vi "Begin.vi"(8 "error in":errorcluster) -> (0 "error out":errorcluster)   [LabVIEW 2020]
doc: "Called before other user functions, this VI is expected to open initial I/O refnums, load in file data, and do all program initialization. Notice that the <B>error out</B> terminal is simply used for data flow. Wiring it to other structures or subVIs ensures that this VI runs first."
uses:
  <vilib>/Rock Robotics/WPI/DriverStation/WPI_DriverStationRobotMode2.ctl
  <vilib>/Rock Robotics/WPI/Joystick/WPI_JoystickDeviceEnum.ctl
  <vilib>/Rock Robotics/WPI/Solenoid/WPI_SolenoidChannel.ctl
  <vilib>/Rock Robotics/SystemInterfaces/DIO/FPGA_DIOPWMChannel.ctl
  <vilib>/Rock Robotics/SystemInterfaces/DIO/FPGA_DIOChannel.ctl
  <vilib>/Rock Robotics/WPI/Encoder/WPI_EncoderType.ctl
  <vilib>/Rock Robotics/WPI/SafetyOutput/WPI_SafetyOutputConfigMenu.ctl
  Robot Global Data.vi
  <vilib>/Rock Robotics/Network Tables/NT Write String Array.vi
  <vilib>/Rock Robotics/WPI/RobotDrive/WPI_RobotDriveOpen4MotorWithExistingMotors.vi
  <vilib>/Rock Robotics/WPI/Solenoid/WPI_SolenoidOpenDouble.vi
  <vilib>/Rock Robotics/WPI/Counter/WPI_CounterDigitalInputToDigitalSource.vi
  <vilib>/Rock Robotics/WPI/RobotDrive/WPI_RobotDriveOpen2MotorWithVictorSPX.vi
  <vilib>/Rock Robotics/SystemInterfaces/spilib/spi_bus.ctl
  <vilib>/Rock Robotics/WPI/Gyro/WPI_GyroXRS450_SPI_Open.vi
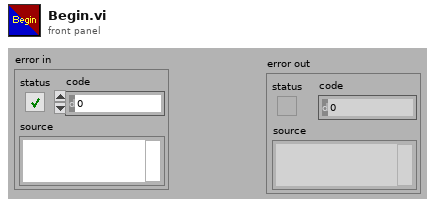
[diagram p1: front panel]
types:
  T1 = typedef "WPI_EncoderType.ctl" = enum16{"1x", "2x", "4x"}
  T2 = typedef "FPGA_DIOChannel.ctl" = enum8{"DIO 0", "DIO 1", "DIO 2", "DIO 3", "DIO 4", "DIO 5", "DIO 6", "DIO 7", "DIO 8", "DIO 9", "DIO MXP 0", "DIO MXP 1", "DIO MXP 2", "DIO MXP 3", "DIO MXP 4", "DIO MXP 5", "DIO MXP 6", "DIO MXP 7", "DIO MXP 8", "DIO MXP 9", "DIO MXP 10", "DIO MXP 11", "DIO MXP 12", "DIO MXP 13", "DIO MXP 14", "DIO MXP 15", "SPI Port CS1", "SPI Port CS2", "SPI Port CS3", "SPI Port MISO", "SPI Port MOSI", "Invalid"}
  T3 = typedef "FPGA_DIOPWMChannel.ctl" = enum8{"PWM 0", "PWM 1", "PWM 2", "PWM 3", "PWM 4", "PWM 5", "PWM 6", "PWM 7", "PWM 8", "PWM 9", "PWM MXP 0", "PWM MXP 1", "PWM MXP 2", "PWM MXP 3", "PWM MXP 4", "PWM MXP 5", "PWM MXP 6", "PWM MXP 7", "PWM MXP 8", "PWM MXP 9", "Invalid"}
  T4 = typedef "WPI_SolenoidChannel.ctl" = enum8{"Solenoid 0", "Solenoid 1", "Solenoid 2", "Solenoid 3", "Solenoid 4", "Solenoid 5", "Solenoid 6", "Solenoid 7", "Solenoid 8", "Solenoid 9", "Solenoid 10", "Solenoid 11", "Solenoid 12", "Solenoid 13", "Solenoid 14", "Solenoid 15", "Invalid"}
  T5 = typedef "WPI_JoystickDeviceEnum.ctl" = enum16{"USB 0", "USB 1", "USB 2", "USB 3", "USB 4", "USB 5"}
  T6 = typedef "WPI_DriverStationRobotMode2.ctl" = enum16{"Autonomous Disabled", "Autonomous Enabled", "Teleop Disabled", "Teleop Enabled", "Disconnected", "Finish", "Test Disabled", "Test Enabled", "Emergency Stopped"}
  T7 = typedef "WPI_MotorControlDeviceRef.ctl" = cluster{"DeviceStatus":errorcluster, "Type":T8, "PWM":cluster{"PWM Channel":T3, "DeadBand":T9}, "CAN":cluster{"Device Number":u8, "SetOutput VI Ref":variant, "GetOutput VI Ref":variant, "Enable VI Ref":variant, "Disable VI Ref":variant, "Data":variant}, "Invert":bool, "DIO PWM":cluster{"PWM \"Enable\" Channel":T3, "DIOChannel":T2, "PWM Rate":dbl}}
  T8 = typedef "WPI_MotorControlType.ctl" = enum16{"PWM", "CAN", "DIO PWM"}
  T9 = typedef "WPI_PWMDeadband.ctl" = cluster{"Name":string, "maxPositivePwm":i32, "minPositivePwm":i32, "centerPwm":i32, "maxNegativePwm":i32, "minNegativePwm":i32, "angularRange":u16}
  T10 = typedef "spi_bus.ctl" = enum16{"SPI On-Board, CS0", "SPI On-Board, CS1", "SPI On-Board, CS2", "SPI On-Board, CS3", "SPI MXP", "Invalid"}
  T11 = typedef "WPI_GyroDevRef.ctl" = cluster{"DevStatus":errorcluster, "Analog Channel":T12, "Gain (VoltsPerDegree/Second)":dbl, "Gyro Type":enum16{"Analog", "XRS450"}, "Handle":i32, "SPI Bus":T10, "Device Found":bool, "Sample Rate":dbl, "Calibrate On Open":bool, "Offset":dbl}
  T12 = typedef "FPGA_AIChannel.ctl" = enum8{"AI 0", "AI 1", "AI 2", "AI 3", "AI MXP 0", "AI MXP 1", "AI MXP 2", "AI MXP 3", "Invalid"}
  T13 = typedef "WPI_ServoDeviceRef.ctl" = cluster{"DeviceStatus":errorcluster, "PWM Channel":T3, "DeadBand":T9}
  T14 = typedef "WPI_JoystickDevRef.ctl" = cluster{"Device":T5}
  T15 = typedef "WPI_DigitalInputDevRef.ctl" = cluster{"DevStatus":errorcluster, "DIO Channel":T2}
  T16 = typedef "FPGA_CounterEncoderSourceConvertionLVSourceType.ctl" = cluster{"DevStatus":errorcluster, "AnalogTriggerMode?":bool, "DigitalMode":cluster{"DIO Channel":T17}, "AnalogTriggerMode":cluster{"AnalogTriggerIndex":T18, "OutputType":T19}}
  T17 = typedef "FPGA_DIODigitalSourceChannel.ctl" = enum8{"DIO 0", "DIO 1", "DIO 2", "DIO 3", "DIO 4", "DIO 5", "DIO 6", "DIO 7", "DIO 8", "DIO 9", "DIO MXP 0", "DIO MXP 1", "DIO MXP 2", "DIO MXP 3", "DIO MXP 4", "DIO MXP 5", "DIO MXP 6", "DIO MXP 7", "DIO MXP 8", "DIO MXP 9", "DIO MXP 10", "DIO MXP 11", "DIO MXP 12", "DIO MXP 13", "DIO MXP 14", "DIO MXP 15", "SPI Port CS1", "SPI Port CS2", "SPI Port CS3", "SPI Port MISO", "SPI Port MOSI", "Disabled"}
  T18 = typedef "FPGA_AnalogTriggerIndex.ctl" = enum8{"Trig 0", "Trig 1", "Trig 2", "Trig 3", "Trig 4", "Trig 5", "Trig 6", "Trig 7", "Invalid"}
  T19 = typedef "FPGA_AnalogTriggerOutType.ctl" = enum16{"InWindow", "TriggerState", "Rising", "Falling"}
  T20 = typedef "WPI_EncoderDevRef.ctl" = cluster{"DevStatus":errorcluster, "EncoderIndex":T21, "CounterIndex":T22, "DistancePerCount":dbl, "Decoding Type":T1}
  T21 = typedef "FPGA_EncoderIdx.ctl" = enum8{"Enc 0", "Enc 1", "Enc 2", "Enc 3", "Enc 4", "Enc 5", "Enc 6", "Enc 7", "Invalid"}
  T22 = typedef "FPGA_CounterCtrSystemIndex.ctl" = enum8{"Ctr 0", "Ctr 1", "Ctr 2", "Ctr 3", "Ctr 4", "Ctr 5", "Ctr 6", "Ctr 7", "Invalid"}
  T23 = typedef "WPI_SafetyOutputConfigMenu.ctl" = enum16{"Enable", "Disable"}
  T24 = typedef "WPI_RobotDriveDevRef.ctl" = cluster{"DevStatus":errorcluster, "Motors[]":T7[], "Square Inputs":bool, "Max Output":dbl}
  T25 = typedef "WPI_SolenoidDevRef.ctl" = cluster{"DevStatus":errorcluster, "Pneumatics Control Module":u8, "Forward Solenoid Channel":T4, "Reverse Solenoid Channel":T4}
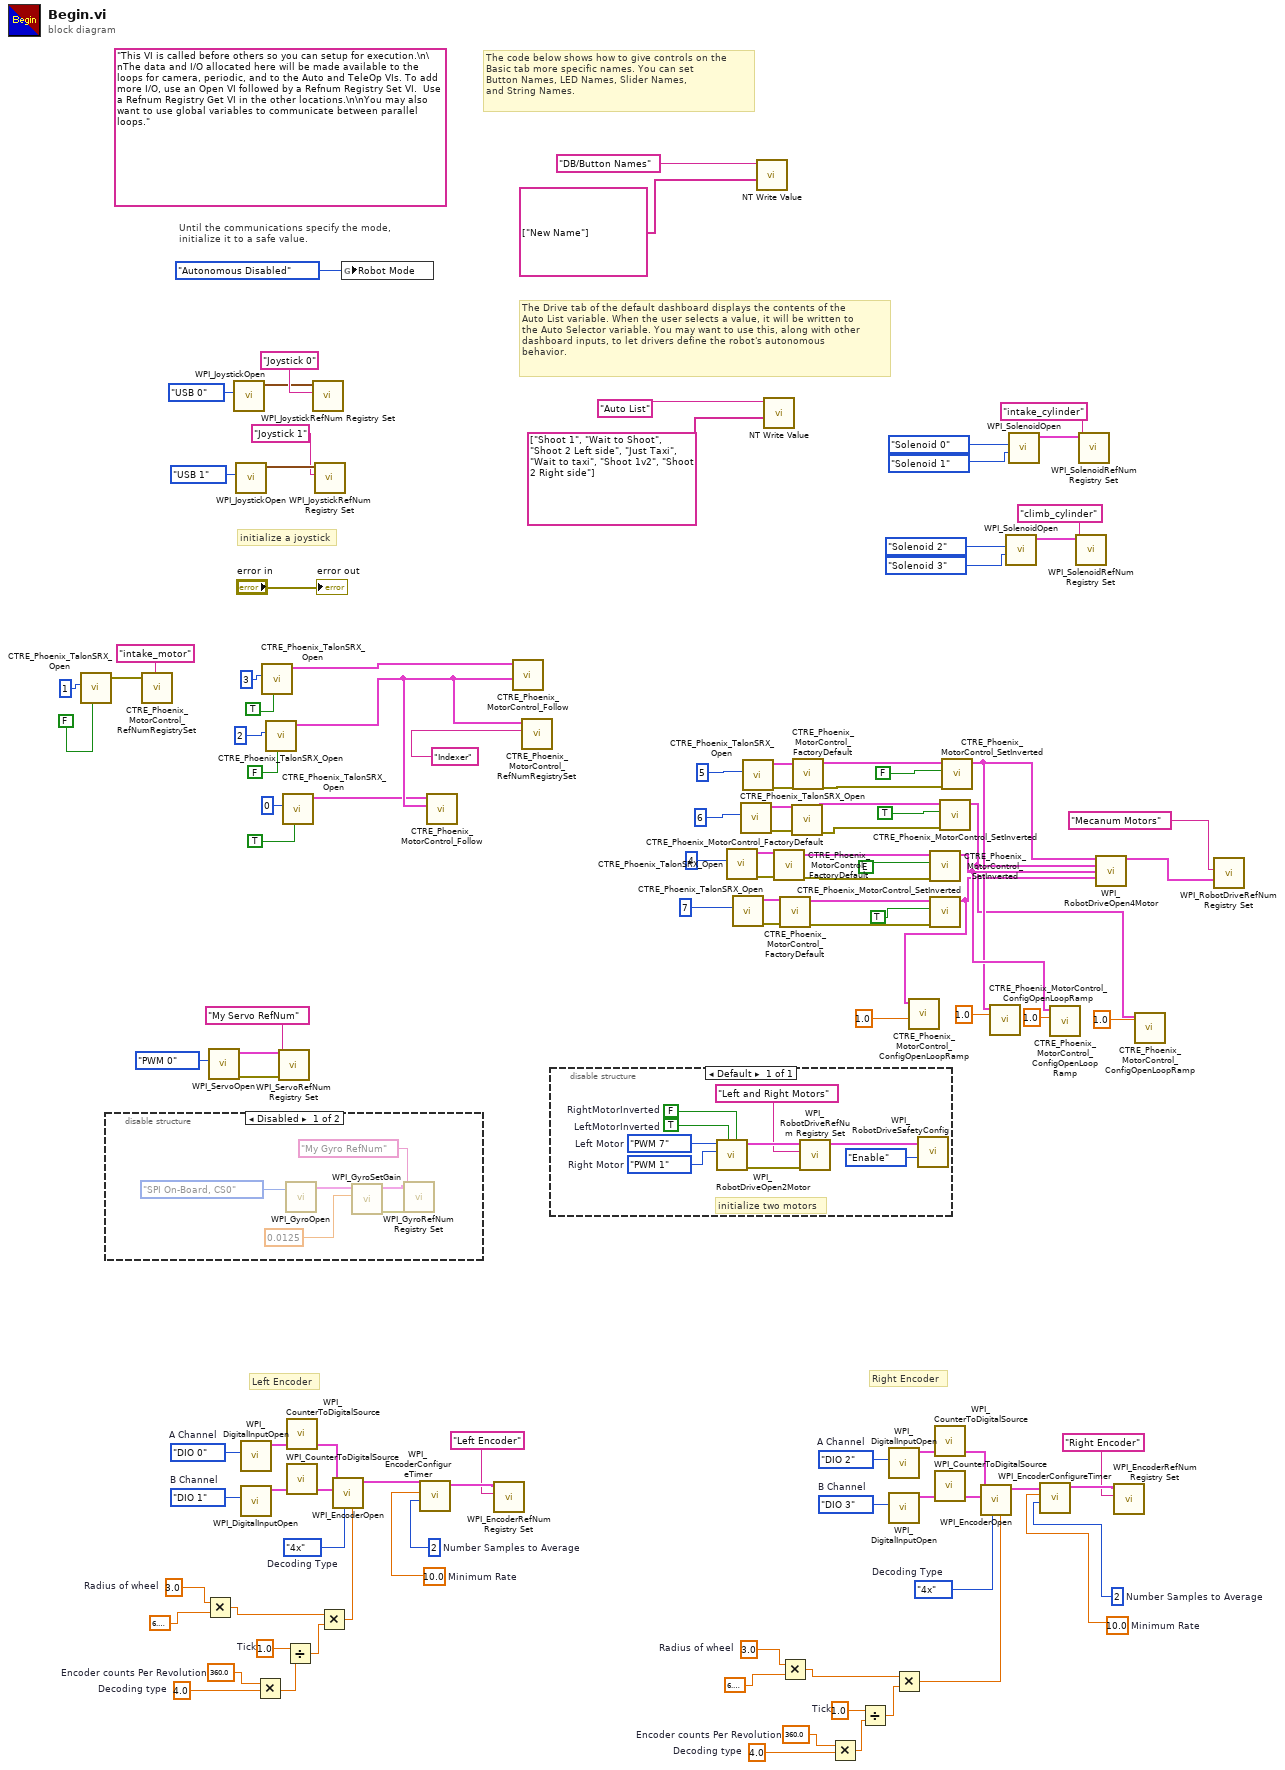
[diagram p0: block diagram]
diagram:
  w5 = u8 2  # Number Samples to Average
  w3 = 10.0  # Minimum Rate
  w9 = 3.0  # Radius of wheel
  w10 = 1.0  # Tick
  w13 = 360.0  # Encoder counts Per Revolution
  w14 = 4.0  # Decoding type
  w6 = WPI_EncoderType."4x"  # Decoding Type
  w1 = u8 2  # Number Samples to Average
  w15 = 10.0  # Minimum Rate
  w17 = 3.0  # Radius of wheel
  w19 = 1.0  # Tick
  w23 = 360.0  # Encoder counts Per Revolution
  w24 = 4.0  # Decoding type
  w2 = WPI_EncoderType."4x"  # Decoding Type
  w34 = FPGA_DIOChannel."DIO 3"  # B Channel
  w33 = FPGA_DIOChannel."DIO 2"  # A Channel
  w40 = FPGA_DIOChannel."DIO 1"  # B Channel
  w39 = FPGA_DIOChannel."DIO 0"  # A Channel
  (unwired) "This VI is called before others so you can setup for execution.\n\nThe data and I/O allocated here will be made available to the loops for camera, periodic, and to the Auto and TeleOp VIs. To add more I/O, use an Open VI followed by a Refnum Registry Set VI.  Use a Refnum Registry Get VI in the other locations.\n\nYou may also want to use global variables to communicate between parallel loops."
  # "Right Encoder"
  # "Left Encoder"
  # "The Drive tab of the default dashboard displays the contents of the\nAuto List variable. When the user selects a value, it will be written to\nthe Auto Selector variable. You may want to use this, along with other\ndashboard inputs, to let drivers define the robot's autonomous\nbehavior."
  # "The code below shows how to give controls on the\nBasic tab more specific names. You can set\nButton Names, LED Names, Slider Names,\nand String Names."
  # "initialize a joystick"
  # "Until the communications specify the mode,\ninitialize it to a safe value."
  n1 = call <vilib>:"CTRE_Phoenix_TalonSRX_Open.vi"("Invert"=FALSE, "Device Number"=u8 1) -> ("error out"=w79:errorcluster, "PhoenixMotorControlDevRef"=w78:T7)  [unwired: 8 in]
  n2 = disable-structure shown="Disabled" {
    frame Disabled {
      n3 = call-poly <vilib>:"WPI_GyroOpen.vi"("SPI Bus"=spi_bus."SPI On-Board, CS0") -> ("GyroDevRef"=w118:T11)  [unwired: 8 in, 2 out]
      n4 = call <vilib>:"WPI_GyroSetGain.vi"("Gain (VoltsPerDegree/Second)"=0.0125, "GyroDevRef"=w118) -> ("error out"=w119:errorcluster, "GyroDevRef"=w117:T11)  [unwired: 8 in]
      n5 = call <vilib>:"WPI_GyroRefNum Registry Set.vi"("error in (no error)"=w119, "refnum name"="My Gyro RefNum", "GyroDevRef"=w117) -> ()  [unwired: 7 in, 2 out]
    }
    frame Enabled {
    }
  }
  n6 = call <vilib>:"CTRE_Phoenix_MotorControl_RefNumRegistrySet.vi"("error in (no error)"=w79, "refnum name"="intake_motor", "PhoenixMotorControlDevRef"=w78) -> ()  [unwired: 7 in, 2 out]
  n7 = Multiply(x=w17, y=6.283185307179586) -> (x*y=w18:dbl)
  n8 = call <vilib>:"WPI_ServoOpen.vi"("PWM Channel"=FPGA_DIOPWMChannel."PWM 0") -> ("error out"=w44:errorcluster, "ServoDeviceRef"=w45:T13)  [unwired: 9 in]
  n9 = call <vilib>:"WPI_JoystickOpen.vi"("JoystickDevice"=WPI_JoystickDeviceEnum."USB 0") -> ("JoystickDevRef"=w112:T14)  [unwired: 10 in]
  n10 = call <vilib>:"WPI_JoystickOpen.vi"("JoystickDevice"=WPI_JoystickDeviceEnum."USB 1") -> ("JoystickDevRef"=w76:T14)  [unwired: 10 in]
  n11 = call <vilib>:"WPI_DigitalInputOpen.vi"("DIO Channel"=w39) -> ("DigitalInputDevRef"=w37:T15)  [unwired: 1 in, 9 out]
  n12 = call <vilib>:"WPI_DigitalInputOpen.vi"("DIO Channel"=w40) -> ("DigitalInputDevRef"=w38:T15)  [unwired: 1 in, 9 out]
  n13 = Multiply(x=w23, y=w24) -> (x*y=w20:dbl)
  n14 = call <vilib>:"CTRE_Phoenix_TalonSRX_Open.vi"("Invert"=TRUE, "Device Number"=u8 3) -> ("PhoenixMotorControlDevRef"=w67:T7)  [unwired: 8 in, 1 out]
  n15 = call <vilib>:"CTRE_Phoenix_TalonSRX_Open.vi"("Invert"=FALSE, "Device Number"=u8 2) -> ("PhoenixMotorControlDevRef"=w48:T7)  [unwired: 8 in, 1 out]
  n16 = call <vilib>:"WPI_ServoRefNum Registry Set.vi"("error in (no error)"=w44, "refnum name"="My Servo RefNum", "ServoDeviceRef"=w45) -> ()  [unwired: 7 in, 2 out]
  n17 = call <vilib>:"CTRE_Phoenix_TalonSRX_Open.vi"("Invert"=TRUE, "Device Number"=u8 0) -> ("PhoenixMotorControlDevRef"=w47:T7)  [unwired: 8 in, 1 out]
  n18 = Divide(x=w19, y=w20) -> (x/y=w21:dbl)
  n19 = call-poly <vilib>:"WPI_CounterToDigitalSource.vi"("DigitalInputDevRef"=w37) -> ("Digital Source"=w41:T16)  [unwired: 6 out]
  n20 = call-poly <vilib>:"WPI_CounterToDigitalSource.vi"("DigitalInputDevRef"=w38) -> ("Digital Source"=w42:T16)  [unwired: 6 out]
  n21 = call <vilib>:"WPI_JoystickRefNum Registry Set.vi"("refnum name"="Joystick 0", "JoystickDevRef"=w112) -> ()  [unwired: 8 in, 2 out]
  n22 = call <vilib>:"WPI_JoystickRefNum Registry Set.vi"("refnum name"="Joystick 1", "JoystickDevRef"=w76) -> ()  [unwired: 8 in, 2 out]
  n23 = Multiply(x=w18, y=w21) -> (x*y=w22:dbl)
  n24 = call <vilib>:"WPI_EncoderOpen.vi"("DistancePerCount"=w22, "Decoding Type"=w2, "BSource"=w42, "ASource"=w41) -> ("EncoderDevRef"=w30:T20)  [unwired: 6 in, 1 out]
  n25 = global write "Robot Global Data.vi" "Robot Mode"(WPI_DriverStationRobotMode2."Autonomous Disabled" ("Robot Mode")) -> ()
  n26 = call <vilib>:"WPI_EncoderConfigureTimer.vi"("Number Samples to Average"=w1, "Minimum Rate"=w15, "EncoderDevRef"=w30) -> ("EncoderDevRef"=w29:T20)  [unwired: 7 in, 1 out]
  n27 = call <vilib>:"CTRE_Phoenix_MotorControl_Follow.vi"("Master Controller to Follow"=w48, "PhoenixMotorControlDevRef"=w47) -> ()  [unwired: 8 in, 2 out]
  n28 = call <vilib>:"WPI_EncoderRefNum Registry Set.vi"("refnum name"="Left Encoder", "EncoderDevRef"=w29) -> ()  [unwired: 8 in, 2 out]
  n29 = call <vilib>:"CTRE_Phoenix_MotorControl_Follow.vi"("Master Controller to Follow"=w48, "PhoenixMotorControlDevRef"=w67) -> ()  [unwired: 8 in, 2 out]
  n30 = call <vilib>:"CTRE_Phoenix_MotorControl_RefNumRegistrySet.vi"("refnum name"="Indexer", "PhoenixMotorControlDevRef"=w48) -> ()  [unwired: 8 in, 2 out]
  n31 = disable-structure shown="Default" {
    frame Enabled {
      w123 = FPGA_DIOPWMChannel."PWM 1"  # Right Motor
      w124 = FPGA_DIOPWMChannel."PWM 7"  # Left Motor
      w128 = TRUE  # LeftMotorInverted
      w129 = FALSE  # RightMotorInverted
      # "initialize two motors"
      n32 = call-poly <vilib>:"WPI_RobotDriveOpen2Motor.vi"("Right Motor Inverted"=w129, "Left Motor Inverted"=w128, "Right Motor"=w123, "Left Motor"=w124) -> ("error out"=w125:errorcluster, "RobotDriveDevRef"=w127:T24)  [unwired: 1 in, 5 out]
      n33 = call <vilib>:"WPI_RobotDriveRefNum Registry Set.vi"("error in (no error)"=w125, "refnum name"="Left and Right Motors", "RobotDriveDevRef"=w127) -> ("RobotDriveDevRef"=w122:T24)  [unwired: 1 in, 7 out]
      n34 = call <vilib>:"WPI_RobotDriveSafetyConfig.vi"("mode"=WPI_SafetyOutputConfigMenu."Enable", "RobotDriveDevRef"=w122) -> ()  [unwired: 8 in, 2 out]
    }
  }
  n35 = call <vilib>:"CTRE_Phoenix_TalonSRX_Open.vi"("Device Number"=u8 4) -> ("error out"=w104:errorcluster, "PhoenixMotorControlDevRef"=w105:T7)  [unwired: 9 in]
  n36 = call <vilib>:"CTRE_Phoenix_TalonSRX_Open.vi"("Device Number"=u8 7) -> ("error out"=w94:errorcluster, "PhoenixMotorControlDevRef"=w95:T7)  [unwired: 9 in]
  n37 = call <vilib>:"CTRE_Phoenix_TalonSRX_Open.vi"("Device Number"=u8 6) -> ("error out"=w98:errorcluster, "PhoenixMotorControlDevRef"=w99:T7)  [unwired: 9 in]
  n38 = call <vilib>:"CTRE_Phoenix_TalonSRX_Open.vi"("Device Number"=u8 5) -> ("error out"=w91:errorcluster, "PhoenixMotorControlDevRef"=w101:T7)  [unwired: 9 in]
  n39 = call-poly <vilib>:"NT Write Value.vi"("String Array"=string[] ["New Name"], "Name"="DB/Button Names") -> ()  [unwired: 9 in, 1 out]
  n40 = call-poly <vilib>:"NT Write Value.vi"("String Array"=string[] ["Shoot 1", "Wait to Shoot", "Shoot 2 Left side", "Just Taxi", "Wait to taxi", "Shoot 1v2", "Shoot 2 Right side"], "Name"="Auto List") -> ()  [unwired: 9 in, 1 out]
  n41 = call <vilib>:"CTRE_Phoenix_MotorControl_FactoryDefault.vi"("error in"=w104, "PhoenixMotorControlDevRef"=w105) -> ("error out"=w102:errorcluster, "PhoenixMotorControlDevRef"=w103:T7)  [unwired: 8 in]
  n42 = call <vilib>:"CTRE_Phoenix_MotorControl_FactoryDefault.vi"("error in"=w94, "PhoenixMotorControlDevRef"=w95) -> ("error out"=w92:errorcluster, "PhoenixMotorControlDevRef"=w93:T7)  [unwired: 8 in]
  n43 = Multiply(x=w9, y=6.283185307179586) -> (x*y=w4:dbl)
  n44 = call <vilib>:"CTRE_Phoenix_MotorControl_FactoryDefault.vi"("error in"=w98, "PhoenixMotorControlDevRef"=w99) -> ("error out"=w96:errorcluster, "PhoenixMotorControlDevRef"=w97:T7)  [unwired: 8 in]
  n45 = call <vilib>:"CTRE_Phoenix_MotorControl_FactoryDefault.vi"("PhoenixMotorControlDevRef"=w101) -> ("PhoenixMotorControlDevRef"=w100:T7)  [unwired: 9 in, 1 out]
  n46 = Multiply(x=w13, y=w14) -> (x*y=w11:dbl)
  n47 = Divide(x=w10, y=w11) -> (x/y=w12:dbl)
  n48 = call <vilib>:"WPI_DigitalInputOpen.vi"("DIO Channel"=w33) -> ("DigitalInputDevRef"=w31:T15)  [unwired: 1 in, 9 out]
  n49 = call <vilib>:"WPI_DigitalInputOpen.vi"("DIO Channel"=w34) -> ("DigitalInputDevRef"=w32:T15)  [unwired: 1 in, 9 out]
  n50 = Multiply(x=w4, y=w12) -> (x*y=w7:dbl)
  n51 = call <vilib>:"CTRE_Phoenix_MotorControl_SetInverted.vi"("error in (no error)"=w102, "Invert?"=FALSE, "PhoenixMotorControlDevRef"=w103) -> ("PhoenixMotorControlDevRef"=w58:T7)  [unwired: 7 in, 1 out]
  n52 = call <vilib>:"CTRE_Phoenix_MotorControl_SetInverted.vi"("error in (no error)"=w92, "Invert?"=TRUE, "PhoenixMotorControlDevRef"=w93) -> ("PhoenixMotorControlDevRef"=w51:T7)  [unwired: 7 in, 1 out]
  n53 = call <vilib>:"CTRE_Phoenix_MotorControl_ConfigOpenLoopRamp.vi"("secondsFromNeutralToFull"=1.0, "PhoenixMotorControlDevRef"=w51) -> ()  [unwired: 8 in, 2 out]
  n54 = call-poly <vilib>:"WPI_CounterToDigitalSource.vi"("DigitalInputDevRef"=w31) -> ("Digital Source"=w35:T16)  [unwired: 6 out]
  n55 = call-poly <vilib>:"WPI_CounterToDigitalSource.vi"("DigitalInputDevRef"=w32) -> ("Digital Source"=w36:T16)  [unwired: 6 out]
  n56 = call <vilib>:"CTRE_Phoenix_MotorControl_SetInverted.vi"("error in (no error)"=w96, "Invert?"=TRUE, "PhoenixMotorControlDevRef"=w97) -> ("PhoenixMotorControlDevRef"=w52:T7)  [unwired: 7 in, 1 out]
  n57 = call <vilib>:"CTRE_Phoenix_MotorControl_SetInverted.vi"("error in (no error)"=w91, "Invert?"=FALSE, "PhoenixMotorControlDevRef"=w100) -> ("PhoenixMotorControlDevRef"=w57:T7)  [unwired: 7 in, 1 out]
  n58 = call <vilib>:"WPI_EncoderOpen.vi"("DistancePerCount"=w7, "Decoding Type"=w6, "BSource"=w36, "ASource"=w35) -> ("EncoderDevRef"=w25:T20)  [unwired: 6 in, 1 out]
  n59 = call <vilib>:"CTRE_Phoenix_MotorControl_ConfigOpenLoopRamp.vi"("secondsFromNeutralToFull"=1.0, "PhoenixMotorControlDevRef"=w57) -> ()  [unwired: 8 in, 2 out]
  n60 = call-poly <vilib>:"WPI_SolenoidOpen.vi"("Reverse Solenoid Channel"=WPI_SolenoidChannel."Solenoid 3" ("Forward Solenoid Channel"), "Forward Solenoid Channel"=WPI_SolenoidChannel."Solenoid 2") -> ("SolenoidDevRef"=w65:T25)  [unwired: 8 in, 1 out]
  n61 = call-poly <vilib>:"WPI_SolenoidOpen.vi"("Reverse Solenoid Channel"=WPI_SolenoidChannel."Solenoid 1" ("Forward Solenoid Channel"), "Forward Solenoid Channel"=WPI_SolenoidChannel."Solenoid 0") -> ("SolenoidDevRef"=w62:T25)  [unwired: 8 in, 1 out]
  n62 = call <vilib>:"WPI_EncoderConfigureTimer.vi"("Number Samples to Average"=w5, "Minimum Rate"=w3, "EncoderDevRef"=w25) -> ("EncoderDevRef"=w27:T20)  [unwired: 7 in, 1 out]
  n63 = call <vilib>:"CTRE_Phoenix_MotorControl_ConfigOpenLoopRamp.vi"("secondsFromNeutralToFull"=1.0, "PhoenixMotorControlDevRef"=w58) -> ()  [unwired: 8 in, 2 out]
  n64 = call <vilib>:"WPI_SolenoidRefNum Registry Set.vi"("refnum name"="climb_cylinder", "SolenoidDevRef"=w65) -> ()  [unwired: 8 in, 2 out]
  n65 = call <vilib>:"WPI_SolenoidRefNum Registry Set.vi"("refnum name"="intake_cylinder", "SolenoidDevRef"=w62) -> ()  [unwired: 8 in, 2 out]
  n66 = call-poly <vilib>:"WPI_RobotDriveOpen4Motor.vi"("Rear Left Motor Dev Ref"=w57, "Rear Right Motor Dev Ref"=w52, "Front Left Motor Dev Ref"=w58, "Front Right Motor Dev Ref"=w51) -> ("RobotDriveDevRef"=w85:T24)  [unwired: 10 in, 1 out]
  n67 = call <vilib>:"WPI_EncoderRefNum Registry Set.vi"("refnum name"="Right Encoder", "EncoderDevRef"=w27) -> ()  [unwired: 8 in, 2 out]
  n68 = call <vilib>:"CTRE_Phoenix_MotorControl_ConfigOpenLoopRamp.vi"("secondsFromNeutralToFull"=1.0, "PhoenixMotorControlDevRef"=w52) -> ()  [unwired: 8 in, 2 out]
  n69 = call <vilib>:"WPI_RobotDriveRefNum Registry Set.vi"("refnum name"="Mecanum Motors", "RobotDriveDevRef"=w85) -> ()  [unwired: 8 in, 2 out]
  "error out" <- "error in"
